vi "Delete Table Data.vi"(8 "error in (no error)":errorcluster, 10 "Table name":string, 11 "Access in":refnum<class "Access.lvclass">) -> (0 "error out":errorcluster, 3 "Access out":refnum<class "Access.lvclass">)   [LabVIEW 2021, in "Database.lvlib" / "Access.lvclass"]
uses:
  Access.lvclass
  Access.lvclass/Access.ctl
  <vilib>/addons/database/Connection.llb/Conn Execute.vi
  <vilib>/addons/database/Recordset.llb/Rec Destroy - Connection.vi
  <vilib>/addons/database/NI_Database_API.lvlib
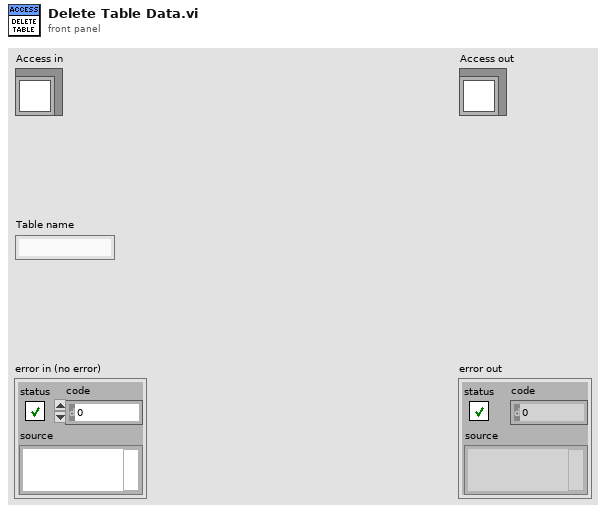
[diagram p1: front panel]
types:
  T1 = typedef "NI_Database_API.lvlib/Conn ObjectReference.ctl" = refnum<k1>
  T2 = typedef "NI_Database_API.lvlib/Rec ObjectReference.ctl" = refnum<k1>
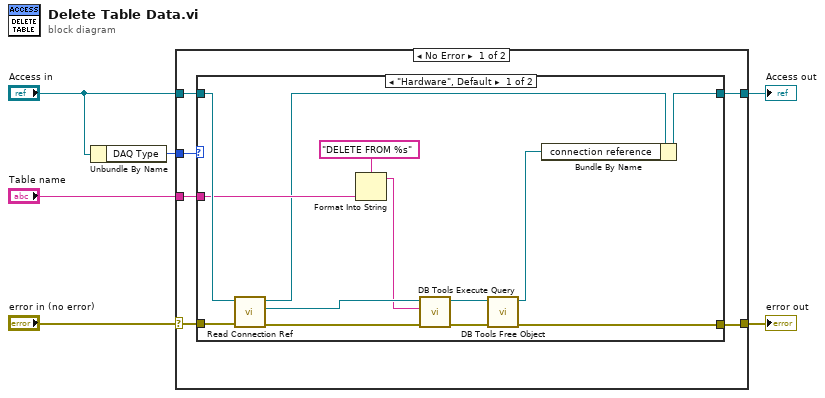
[diagram p0: block diagram]
diagram:
  n1 = Unbundle By Name("Access in") -> ("DAQ Type"=w1:enum16{"Hardware", "Simulation"})
  n2 = case shown="No Error" "error in (no error)" {
    selector: "error in (no error)" -> [w12 w28]
    tunnel: "Access in" -> [w11 w29]
    tunnel: [w10 w29] -> w5
    tunnel: [w9 w28] -> w4
    tunnel: "Table name" -> [w8 _]
    tunnel: w1 -> [w7 _]
    frame No Error {
      n3 = case shown="\"Hardware\", Default" w7 {
        tunnel: w12 -> [w25 w26]
        tunnel: w11 -> [w24 w27]
        tunnel: [w23 w27] -> w10
        tunnel: [w15 w26] -> w9
        tunnel: w8 -> [w14 _]
        frame "Hardware", Default {
          n4 = call-dynamic "Read Connection Ref.vi"("error in (no error)"=w25, "Access in"=w24) -> ("error out"=w22:errorcluster, "connection reference"=w21:T1, "Access out"=w13:refnum<class "Access.lvclass">)  [unwired: 7 in]
          n5 = Format Into String(format string="DELETE FROM %s", w14) -> (resulting string=w19:string)  [unwired: 2 in, 1 out]
          n6 = call-poly <vilib>:"DB Tools Execute Query.vi"("error in (no error)"=w22, "SQL query"=w19, "connection reference"=w21) -> ("error out"=w16:errorcluster, "recordset reference"=w17:T2)  [unwired: 5 in]
          n7 = call-poly <vilib>:"DB Tools Free Object.vi"("error in (no error)"=w16, "recordset reference"=w17) -> ("error out"=w15:errorcluster, "connection reference"=w18:T1)  [unwired: 8 in]
          n8 = Bundle By Name(cluster=w13, "connection reference"=w18) -> (w23:refnum<class "Access.lvclass">)
        }
        frame "Simulation" {
        }
      }
    }
    frame Error {
    }
  }
  "error out" <- w4
  "Access out" <- w5
